vi "BackProp.vi"(0 "Current Layer":dbl[](array[numeric]), 5 "Previous Layer":dbl[](array[numeric]), 7 "NetError":dbl[](array[numeric]), 9 "weights":dbl[](array[numeric]), 11 "PreviousWeights":dbl[](array[numeric]), 13 "Target":dbl[](array[numeric])) -> (4 "w+":dbl[](array[numeric]), 6 "dE_dNET":dbl[](array[numeric]))   [LabVIEW 2014]
panel:
  out "dE_dWi":dbl[](array[numeric])
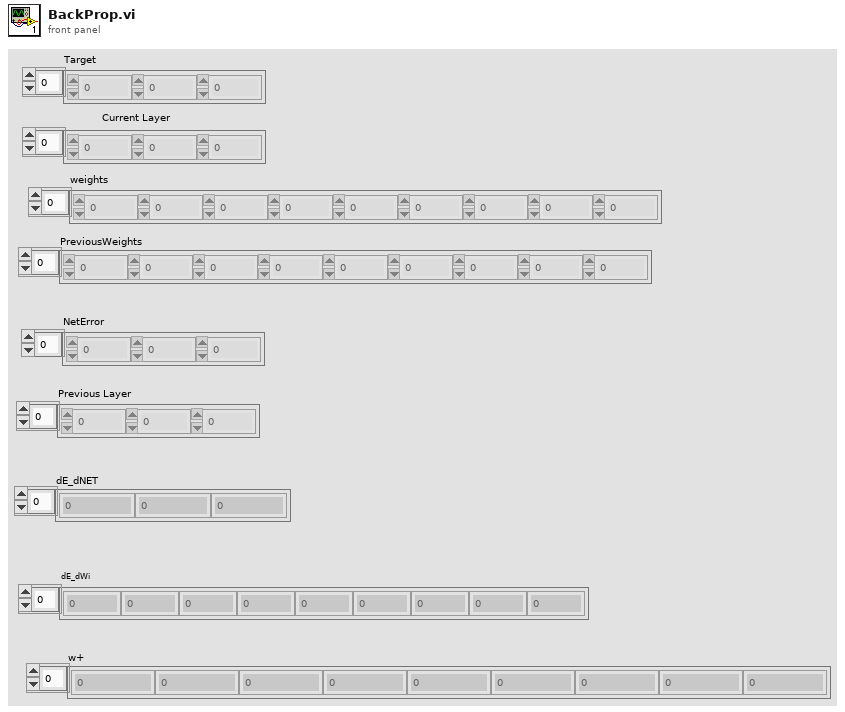
[diagram p1: front panel]
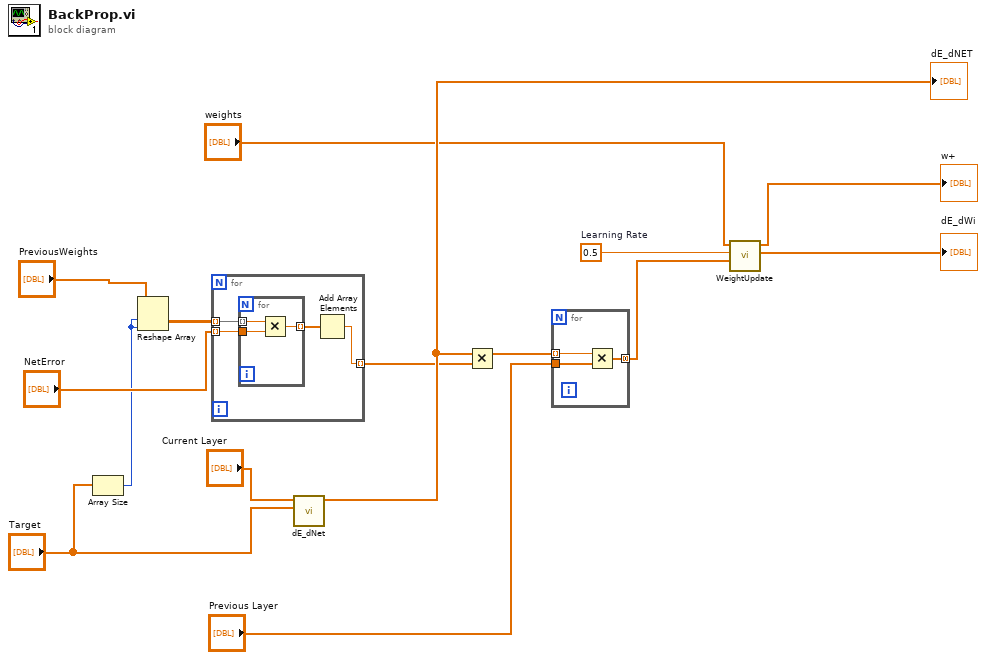
[diagram p0: block diagram]
diagram:
  w14 = 0.5  # Learning Rate
  n1 = Array Size(array="Target") -> (size(s)=w1:i32)
  n2 = Reshape Array("PreviousWeights", w1, w1) -> (w3:dbl[][])
  n3 = for {
    tunnel: w3 -> [w18] mode=indexing
    tunnel: "NetError" -> [w17] mode=indexing
    tunnel: [w16] -> w4 mode=indexing
    n4 = for {
      tunnel: [w22] -> w19 mode=indexing
      tunnel: w18 -> [w21] mode=indexing
      tunnel: w17 -> [w20]
      n5 = Multiply(x=w21, y=w20) -> (x*y=w22:dbl)
    }
    n6 = Add Array Elements(numeric array=w19) -> (sum=w16:dbl)
  }
  n7 = call "dE_dNet.vi"("Target"="Target", "Curren Layer OP"="Current Layer") -> ("dE/dNet"=w15:dbl[])  [unwired: 9 in]
  "dE_dNET" <- w15
  n8 = Multiply(x=w15, y=w4) -> (x*y=w7:dbl[])
  n9 = for {
    tunnel: w7 -> [w25] mode=indexing
    tunnel: "Previous Layer" -> [w24]
    tunnel: [w23] -> w11 mode=concatenating
    n10 = Multiply(x=w25, y=w24) -> (x*y=w23:dbl[])
  }
  n11 = call "WeightUpdate.vi"("(dE/dOut)(PrevLayerOP)"=w11, "Learning Rate"=w14, "weights"="weights") -> ("dE/dWi"=→"dE_dWi":dbl[], "w+"=→"w+":dbl[])  [unwired: 7 in]
